vi "next pattern frame.vi"(10 "Effect":T1(ring)) -> (2 "Array":u16[](array[numeric]))   [LabVIEW 2026]
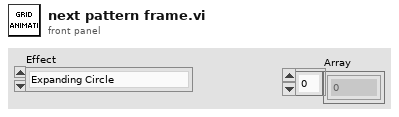
[diagram p1: front panel]
types:
  T1 = enum16{"Expanding Circle", "Plasma", "Radar Sweep", "Matrix Rain", "Campfire", "Diagonal Scan"}
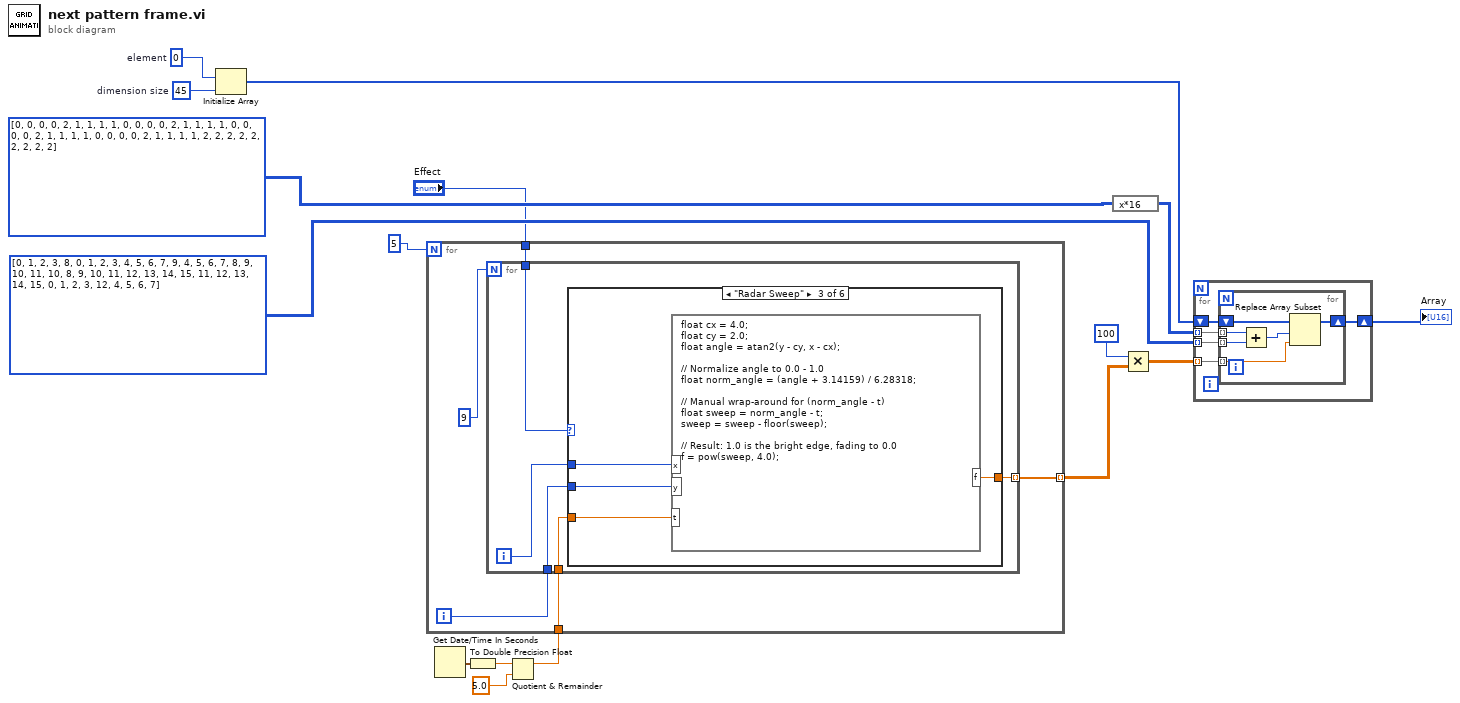
[diagram p0: block diagram]
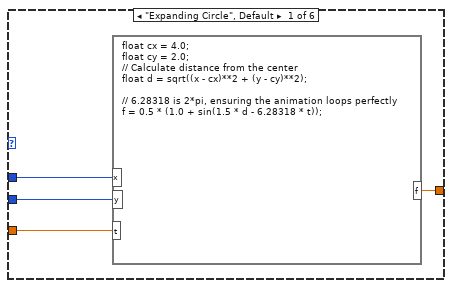
[diagram p2: hidden frame]
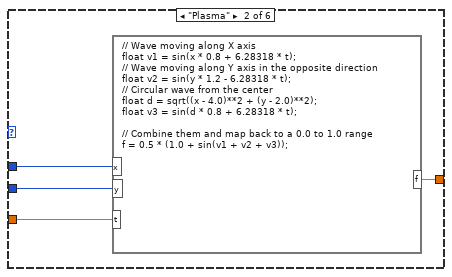
[diagram p3: hidden frame]
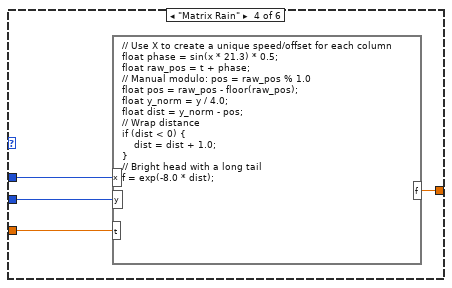
[diagram p4: hidden frame]
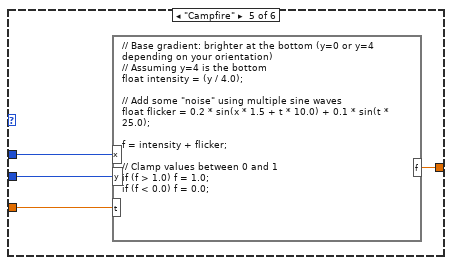
[diagram p5: hidden frame]
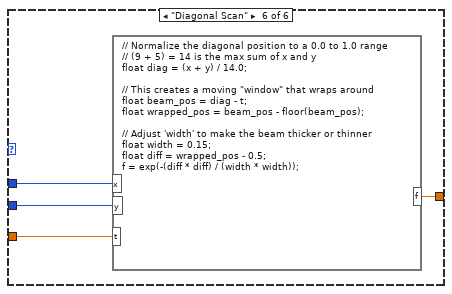
[diagram p6: hidden frame]
diagram:
  w15 = u16 0  # element
  w16 = 45  # dimension size
  n1 = Initialize Array(w15, w16) -> (w14:u16[])
  n2 = Get Date/Time In Seconds() -> (seconds since 1Jan1904=w10:timestamp)
  n3 = To Double Precision Float(number=w10) -> (double precision float=w9:dbl)
  n4 = Quotient & Remainder(x=w9, y=5.0) -> (x-y*floor(x/y)=w7:dbl)  [unwired: 1 out]
  n5 = for {
    N: 5 -> [_]
    tunnel: w7 -> [w19]
    tunnel: [w18] -> w5 mode=indexing
    tunnel: "Effect" -> [w17]
    i -> [w20]
    n6 = for {
      N: 9 -> [_]
      tunnel: w20 -> [w25]
      tunnel: w19 -> [w24]
      tunnel: [w23] -> w18 mode=indexing
      tunnel: w17 -> [w22]
      i -> [w26]
      n7 = case shown="\"Radar Sweep\"" w22 {
        tunnel: w26 -> [w30 w34 w38 w42 w46 w50]
        tunnel: w25 -> [w29 w33 w37 w41 w45 w49]
        tunnel: w24 -> [w28 w32 w36 w40 w44 w48]
        tunnel: [w27 w31 w35 w39 w43 w47] -> w23
        frame "Expanding Circle", Default {
          n8 = formula code="float cx = 4.0;\nfloat cy = 2.0;\n// Calculate distance from the center\nfloat d = sqrt((x - cx)**2 + (y - cy)**2);\n\n// 6.28318 is 2*pi, ensuring the animation loops perfectly\nf = 0.5 * (1.0 + sin(1.5 * d - 6.28318 * t));"("x"=w30, "y"=w29, "t"=w28) -> ("f"=w27:dbl)
        }
        frame "Plasma" {
          n9 = formula code="// Wave moving along X axis\nfloat v1 = sin(x * 0.8 + 6.28318 * t);\n// Wave moving along Y axis in the opposite direction\nfloat v2 = sin(y * 1.2 - 6.28318 * t);\n// Circular wave from the center\nfloat d = sqrt((x - 4.0)**2 + (y - 2.0)**2);\nfloat v3 = sin(d * 0.8 + 6.28318 * t);\n\n// Combine them and map back to a 0.0 to 1.0 range\nf = 0.5 * (1.0 + sin(v1 + v2 + v3));"("x"=w34, "y"=w33, "t"=w32) -> ("f"=w31:dbl)
        }
        frame "Radar Sweep" {
          n10 = formula code="float cx = 4.0;\nfloat cy = 2.0;\nfloat angle = atan2(y - cy, x - cx);\n\n// Normalize angle to 0.0 - 1.0\nfloat norm_angle = (angle + 3.14159) / 6.28318;\n\n// Manual wrap-around for (norm_angle - t)\nfloat sweep = norm_angle - t;\nsweep = sweep - floor(sweep); \n\n// Result: 1.0 is the bright edge, fading to 0.0\nf = pow(sweep, 4.0);"("x"=w38, "y"=w37, "t"=w36) -> ("f"=w35:dbl)
        }
        frame "Matrix Rain" {
          n11 = formula code="// Use X to create a unique speed/offset for each column\nfloat phase = sin(x * 21.3) * 0.5; \nfloat raw_pos = t + phase;\n// Manual modulo: pos = raw_pos % 1.0\nfloat pos = raw_pos - floor(raw_pos);\nfloat y_norm = y / 4.0;\nfloat dist = y_norm - pos;\n// Wrap distance\nif (dist < 0) {\n    dist = dist + 1.0;\n}\n// Bright head with a long tail\nf = exp(-8.0 * dist);"("x"=w42, "y"=w41, "t"=w40) -> ("f"=w39:dbl)
        }
        frame "Campfire" {
          n12 = formula code="// Base gradient: brighter at the bottom (y=0 or y=4 depending on your orientation)\n// Assuming y=4 is the bottom\nfloat intensity = (y / 4.0);\n\n// Add some \"noise\" using multiple sine waves\nfloat flicker = 0.2 * sin(x * 1.5 + t * 10.0) + 0.1 * sin(t * 25.0);\n\nf = intensity + flicker;\n\n// Clamp values between 0 and 1\nif (f > 1.0) f = 1.0;\nif (f < 0.0) f = 0.0;"("x"=w46, "y"=w45, "t"=w44) -> ("f"=w43:dbl)
        }
        frame "Diagonal Scan" {
          n13 = formula code="// Normalize the diagonal position to a 0.0 to 1.0 range\n// (9 + 5) = 14 is the max sum of x and y\nfloat diag = (x + y) / 14.0; \n\n// This creates a moving \"window\" that wraps around\nfloat beam_pos = diag - t;\nfloat wrapped_pos = beam_pos - floor(beam_pos);\n\n// Adjust 'width' to make the beam thicker or thinner\nfloat width = 0.15;\nfloat diff = wrapped_pos - 0.5;\nf = exp(-(diff * diff) / (width * width));"("x"=w50, "y"=w49, "t"=w48) -> ("f"=w47:dbl)
        }
      }
    }
  }
  n14 = expression code="x*16"(i32[][] [[0, 0, 0, 0, 2, 1, 1, 1, 1], [0, 0, 0, 0, 2, 1, 1, 1, 1], [0, 0, 0, 0, 2, 1, 1, 1, 1], [0, 0, 0, 0, 2, 1, 1, 1, 1], [2, 2, 2, 2, 2, 2, 2, 2, 2]]) -> (w2:i32[][])
  n15 = Multiply(x=100, y=w5) -> (x*y=w4:dbl[][])
  n16 = for {
    shift-right: [w54] -> w1
    shift-left: w14 -> [w55]
    tunnel: w4 -> [w53] mode=indexing
    tunnel: w2 -> [w52] mode=indexing
    tunnel: i32[][] [[0, 1, 2, 3, 8, 0, 1, 2, 3], [4, 5, 6, 7, 9, 4, 5, 6, 7], [8, 9, 10, 11, 10, 8, 9, 10, 11], [12, 13, 14, 15, 11, 12, 13, 14, 15], [0, 1, 2, 3, 12, 4, 5, 6, 7]] -> [w51] mode=indexing
    n17 = for {
      shift-right: [w60] -> w54
      shift-left: w55 -> [w61]
      tunnel: w53 -> [w59] mode=indexing
      tunnel: w52 -> [w58] mode=indexing
      tunnel: w51 -> [w57] mode=indexing
      n18 = Add(x=w58, y=w57) -> (x+y=w56:i32)
      n19 = Replace Array Subset(array=w61, new element=w59, index=w56) -> (w60:u16[])
    }
  }
  "Array" <- w1
